vi "enumerateStaticDependencies.vi"(8 "error in (no error)":errorcluster, 11 "System":refnum<class "System.lvclass">) -> (0 "error out":errorcluster, 2 "Static Dependencies":refnum<class "Dependency.lvclass">[](array[class]), 3 "System out":refnum<class "System.lvclass">)   [LabVIEW 2014, in "System.lvclass"]
doc: "JKI State Machine Objects (SMO) 1.4.0.57\nJKI - JKI\nCopyright (c) 2018, JKI"
uses:
  System.lvclass
  <vilib>/JKI/JKI SMO/Dependency/Dependency.lvclass
  Pump.Simulated class/Pump.Simulated.lvclass
  <vilib>/JKI/JKI SMO/SMO/SMO.lvclass
panel:
  # "For instructions on how to use the JKI State Machine Objects, examples and video tutorials, visit:\nhttp://jki.net/state-machine-objects/\n\nJKI State Machine Objects™\nhttp://jki.net/state-machine-objects/\nCopyright (C) 2005-2015, JKI <info@jki.net>\nALL RIGHTS RESERVED"
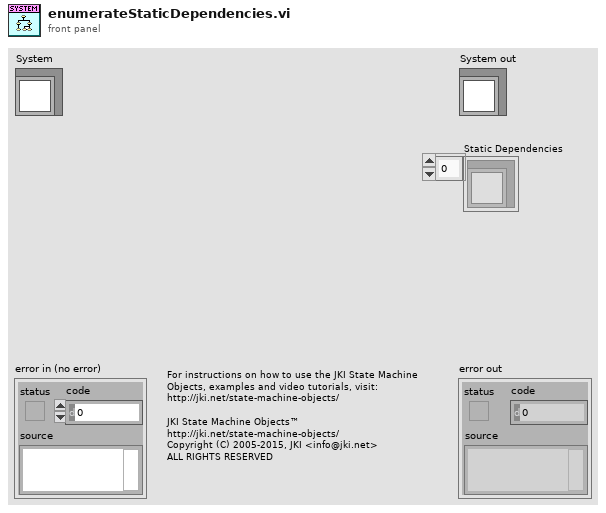
[diagram p1: front panel]
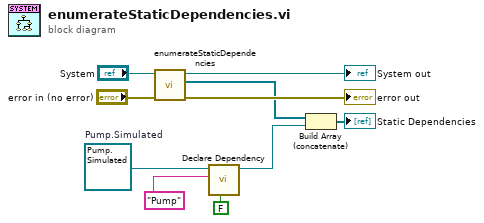
[diagram p0: block diagram]
diagram:
  w1 = refnum<class "Pump.Simulated.lvclass"> refnum  # Pump.Simulated
  n1 = call-parent "enumerateStaticDependencies.vi"("error in (no error)"="error in (no error)", "SMO"="System") -> ("error out"=→"error out":errorcluster, "Static Dependencies"=w3:refnum<class "Dependency.lvclass">[], "SMO out"=→"System out":refnum<class "System.lvclass">)  [unwired: 7 in]
  n2 = call <vilib>:"Declare Dependency.vi"("Shared Resource (F)"=FALSE, "Name"="Pump", "Type"=w1) -> ("Dependency out"=w4:refnum<class "Dependency.lvclass">)  [unwired: 7 in, 1 out]
  n3 = Build Array (concatenate)(w3, w4) -> (→"Static Dependencies":refnum<class "Dependency.lvclass">[])
